vi "ReadHoldingRegs.vi"(8 "error in (no error)":errorcluster, 9 "Config":T1, 11 "Hardware Resources in":T3) -> (0 "error out":errorcluster, 1 "output cluster":T1, 3 "Hardware Resources out":T3)   [LabVIEW 2016]
uses:
  Hardware Configuration.ctl
  Settings/Settings.ctl
  Logging/Logging Configuration.ctl
  Acquisition.lvlib
  Logging/Logging.lvlib
  Settings/Settings.lvlib
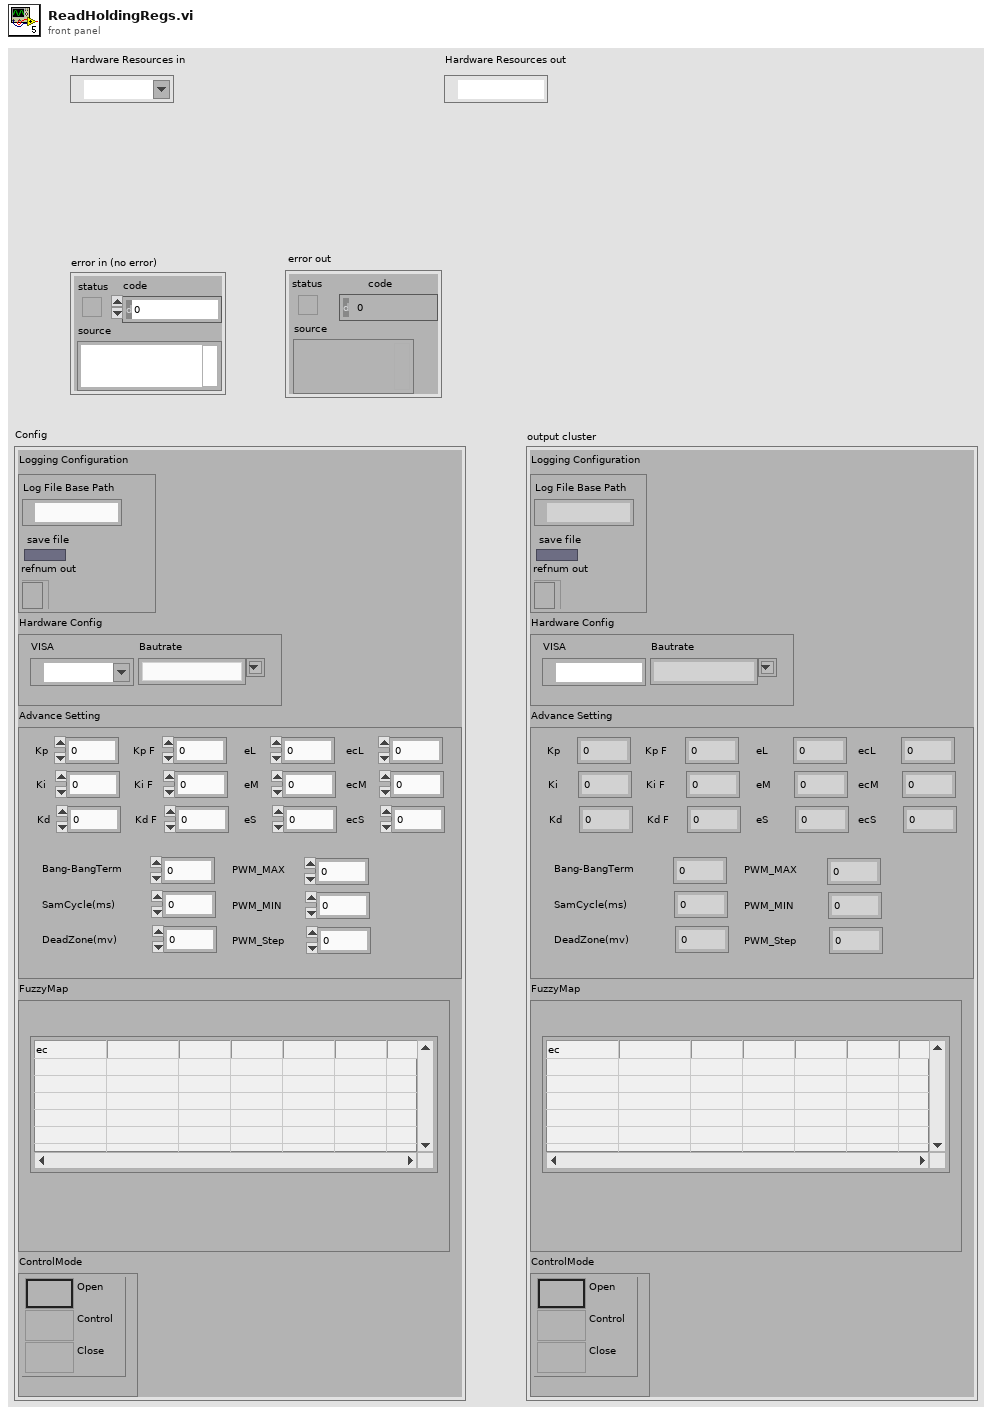
[diagram p1: front panel]
types:
  T1 = typedef "Settings.lvlib/Settings.ctl" = cluster{"Logging Configuration":T2, "Hardware Config":cluster{"Bautrate":string, "VISA":T3}, "Advance Setting":cluster{"PWM_Step":dbl, "PWM_MIN":dbl, "PWM_MAX":dbl, "DeadZone(mv)":dbl, "SamCycle(ms)":dbl, "Bang-BangTerm":dbl, "ecS":dbl, "ecM":dbl, "ecL":dbl, "eS":dbl, "eM":dbl, "eL":dbl, "Kd F":dbl, "Ki F":dbl, "Kp F":dbl, "Kd":dbl, "Ki":dbl, "Kp":dbl}, "FuzzyMap":cluster{"Table":string[][]}, "ControlMode":cluster{"Control":enum32{"1", "2", "4"}}}
  T2 = typedef "Logging.lvlib/Logging Configuration.ctl" = cluster{"Log File Base Path":path, "save file":bool, "refnum out":refnum<file>}
  T3 = typedef "Acquisition.lvlib/Hardware Configuration.ctl" = refnum<visa-resource-name>
  T4 = cluster{"[0]":i32, "[1]":i32, "[2]":i32, "[3]":i32, "[4]":i32, "[5]":i32, "[6]":i32, "[7]":i32, "[8]":i32, "[9]":i32, "[10]":i32, "[11]":i32, "[12]":i32, "[13]":i32, "[14]":i32, "[15]":i32, "[16]":i32, "[17]":i32}
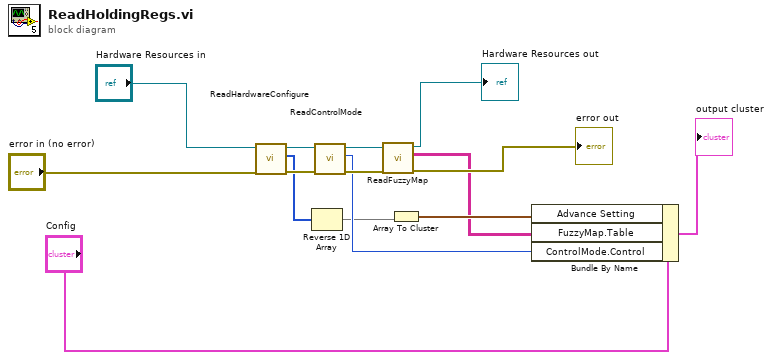
[diagram p0: block diagram]
diagram:
  n1 = call "ReadHardwareConfigure.vi"("error in (no error)"="error in (no error)", "Hardware Resources in"="Hardware Resources in") -> ("error out"=w9:errorcluster, "Output Registers"=w1:i32[], "Hardware Resources out"=w14:T3)  [unwired: 7 in]
  n2 = Reverse 1D Array(array=w1) -> (reversed array=w2:i32[])
  n3 = call "ReadControlMode.vi"("error in (no error)"=w9, "Hardware Resources in"=w14) -> ("error out"=w8:errorcluster, "number"=w3:u32, "Hardware Resources out"=w13:T3)  [unwired: 7 in]
  n4 = call "ReadFuzzyMap.vi"("error in (no error)"=w8, "VISA in"=w13) -> ("error out"=→"error out":errorcluster, "Table Control"=w4:string[][], "VISA out"=→"Hardware Resources out":refnum<visa-resource-name>)  [unwired: 6 in]
  n5 = Array To Cluster(array=w2) -> (cluster=w5:T4)
  n6 = Bundle By Name(cluster="Config", "Advance Setting"=w5, "FuzzyMap.Table"=w4, "ControlMode.Control"=w3) -> (→"output cluster":T1)
